vi "Get EventTypeID.vi"(8 "error in (no error)":errorcluster, 11 "EventToken in":refnum<class "EventToken.lvclass">) -> (0 "error out":errorcluster, 2 "EventData Class":refnum<class "EventData.lvclass">, 3 "EventToken out":refnum<class "EventToken.lvclass">)   [LabVIEW 2009, in "EventManagerLibrary.lvlib" / "EventToken.lvclass"]
uses:
  EventToken.lvclass
  EventDataObject/EventData.lvclass
  EventToken.lvclass/EventToken.ctl
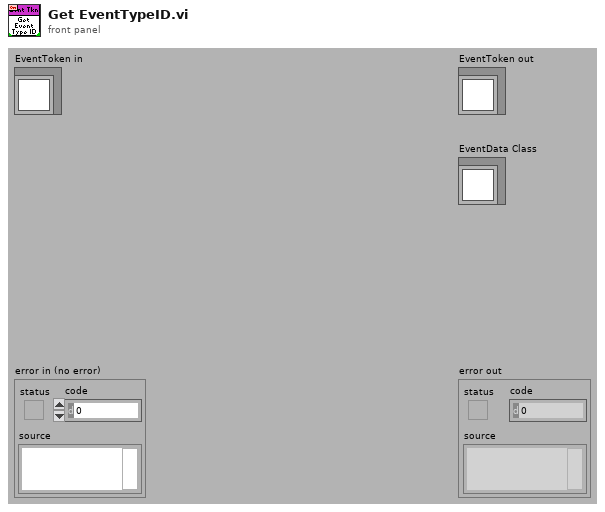
[diagram p1: front panel]
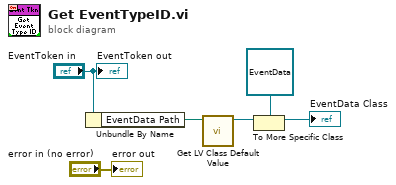
[diagram p0: block diagram]
diagram:
  n1 = Unbundle By Name("EventToken in") -> ("EventData Path"=w4:path)
  n2 = call <vilib>:"Get LV Class Default Value.vi"("class path"=w4) -> ("object"=w3:refnum<class>)  [unwired: 1 in, 9 out]
  n3 = To More Specific Class(target class=refnum<class "EventData.lvclass"> refnum ("EventData Class"), reference=w3) -> (specific class reference=→"EventData Class":refnum<class "EventData.lvclass">)  [unwired: 1 in, 1 out]
  "error out" <- "error in (no error)"
  "EventToken out" <- "EventToken in"
